vi "Rec Fetch Next Recordset (R).vi"(4 "error in (no error)":errorcluster, 7 "recordset reference":T1) -> (0 "error out":errorcluster, 3 "recordset reference out":T1)   [LabVIEW 2013, in "NI_Database_API_64.lvlib"]
doc: "Retrieves the next recordset in a multi-recordset query identified by <B>recordset reference</B>. When the current recordset is no longer available, the <B>recordset reference</B> is redirected to the new recordset. Wire data to the reference input to determine the polymorphic instance to use or manually select the instance."
uses:
  NI_Database_API_64.lvlib
  Rec ObjectReference.ctl
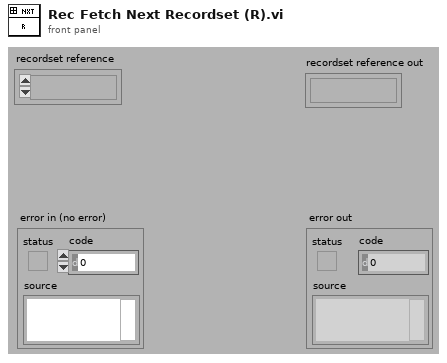
[diagram p1: front panel]
types:
  T1 = typedef "NI_Database_API_64.lvlib/Rec ObjectReference.ctl" = refnum<k1>
  T2 = typedef "NI_Database_API_64.lvlib/Rec DataMembers.ctl" = cluster{"ADODB._Recordset":refnum<k7>, "Connection":T3}
  T3 = typedef "NI_Database_API_64.lvlib/Conn ObjectReference.ctl" = refnum<k1>
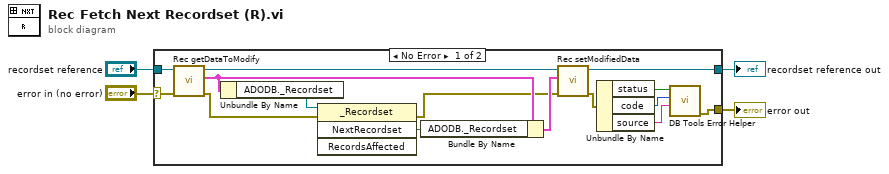
[diagram p0: block diagram]
diagram:
  n1 = case shown="No Error" "error in (no error)" {
    selector: "error in (no error)" -> [w5 w21]
    tunnel: "recordset reference" -> [w18 w20]
    tunnel: [w11 w20] -> w3
    tunnel: [w6 w21] -> w2
    frame No Error {
      n2 = call "Rec getDataToModify.vi"("error in (no error)"=w5, "recordset reference"=w18) -> ("error out"=w15:errorcluster, "data"=w19:T2, "recordset reference out"=w12:T1)  [unwired: 3 out]
      n3 = Unbundle By Name(w19) -> ("ADODB._Recordset"=w16:refnum<k7>)
      n4 = invoke class="_Recordset" method="NextRecordset"(reference=w16, error in=w15) -> (error out=w13:errorcluster, "NextRecordset"=w14:refnum<k7>)  [unwired: 2 in, 2 out]
      n5 = Bundle By Name(cluster=w19, "ADODB._Recordset"=w14) -> (w17:T2)
      n6 = call "Rec setModifiedData.vi"("error in (no error)"=w13, "data"=w17, "recordset reference"=w12) -> ("error out"=w7:errorcluster, "recordset reference out"=w11:T1)  [unwired: 3 out]
      n7 = Unbundle By Name(w7) -> ("status"=w9:bool, "code"=w8:i32, "source"=w10:string)
      n8 = call "DB Tools Error Helper.vi"("source"=w10, "code"=w8, "status"=w9) -> ("error out"=w6:errorcluster)  [unwired: 1 in, 7 out]
    }
    frame Error {
    }
  }
  "recordset reference out" <- w3
  "error out" <- w2
